vi "Exercise 4.2 Debug WebCam on Display.vi"() -> ()   [LabVIEW 2014]
uses:
  <vilib>/Q-Wave Systems/QwaveSys RPi Training Package (Demo)/Addons/QwaveSys RPi Training Library.lvlib
panel:
  in  "Image Size":T1(ring)
  in  "camnum":i32
  out "h":i32
  out "w":i32
  in  "stop":bool
  out "return type 2":i32
  out "return type":i32
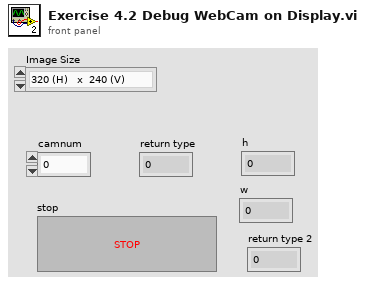
[diagram p1: front panel]
types:
  T1 = enum16{"320 (H)   x  240 (V)", "352(H)    x  288 (V)", "640 (H)   x  480 (V) ", "800 (H)   x  600 (V)", "1024 (H) x  768 (V)", "1280 (H) x  720 (V)", "1280 (H) x 1024 (V)", "1920 (H) x 1080 (V)"}
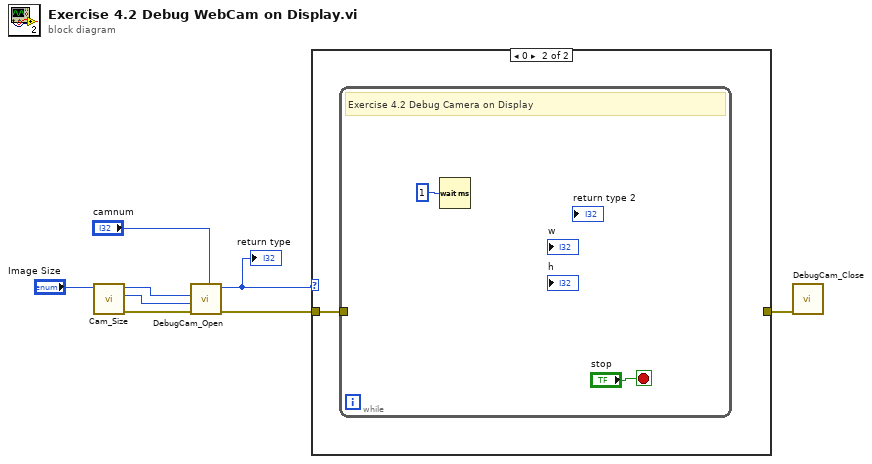
[diagram p0: block diagram]
diagram:
  n1 = call <vilib>:"Cam_Size.vi"("Image Size"="Image Size") -> ("error out"=w5:errorcluster, "h"=w2:i32, "w"=w3:i32)  [unwired: 8 in]
  n2 = call <vilib>:"DebugCam_Open.vi"("error in (no error)"=w5, "h"=w2, "w"=w3, "camnum"="camnum") -> ("error out"=w7:errorcluster, "status"=w1:i32)  [unwired: 6 in]
  "return type" <- w1
  n3 = case shown="0" w1 {
    tunnel: w7 -> [w9 w10]
    tunnel: [w9 _] -> w6
    frame -1, Default {
    }
    frame 0 {
      n4 = while {
        tunnel: w10 -> [_]
        stop <- "stop" stop-if-true
        # "Exercise 4.2 Debug Camera on Display"
        n5 = Wait (ms)(milliseconds to wait=u32 1) -> ()  [unwired: 1 out]
      }
    }
  }
  n6 = call <vilib>:"DebugCam_Close.vi"("error in (no error)"=w6) -> ()  [unwired: 10 in, 1 out]
